vi "Colonoscopy competition - blank subVI.vi"(0 "Switch A Latched":bool=TRUE, 5 "dt in sec":dbl, 7 "Potentiometer bias (-1 to +1)":dbl, 9 "Encoder 1 count":i64, 11 "Encoder 2 count":i64, 12 "Motor steps 1":i64, 13 "Motor steps 2":i64, 14 "Elapsed Time Out (S)":dbl) -> (4 "Stop":bool, 6 "Motor 1 command":i8=-1, 8 "Motor 2 command":i8=1, 10 "MS lines":bool[](array[boolean]))   [LabVIEW 2016]
panel:
  # "Outputs"
  # "Inputs"
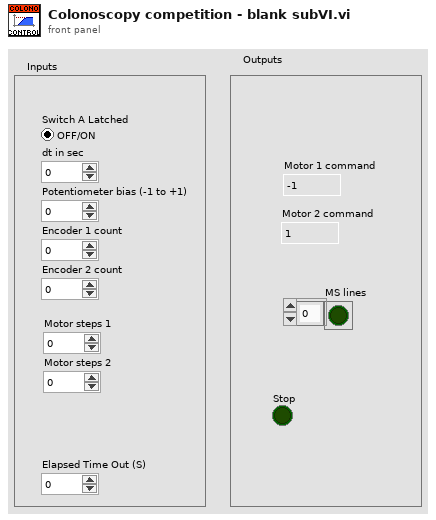
[diagram p1: front panel]
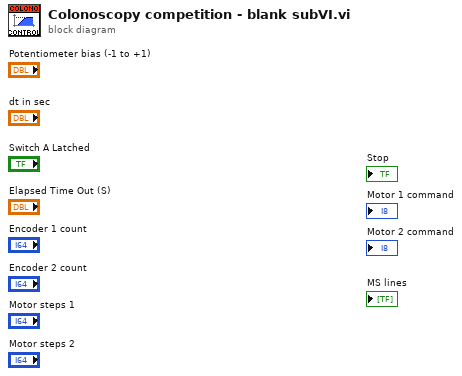
[diagram p0: block diagram]
diagram:
